vi "WaitOnSync.vi"(8 "error in (no error)":errorcluster, 9 "Enable":bool=TRUE, 11 "ControlState in":T1 {"ChainMask" format="0x%02x"}) -> (0 "error out":errorcluster, 3 "ControlState out":T1 {"ChainMask" format="0x%02x"})   [LabVIEW 2023, in "ArduinoSerialBling.lvlib"]
uses:
  ArduinoSerialBling.lvlib
  ControlState.ctl
  ConnectionType.ctl
  UdpConnection.ctl
  ChainState.ctl
  <vilib>/Instr/_visa.llb/VISA Flush IO Buffer Mask.ctl
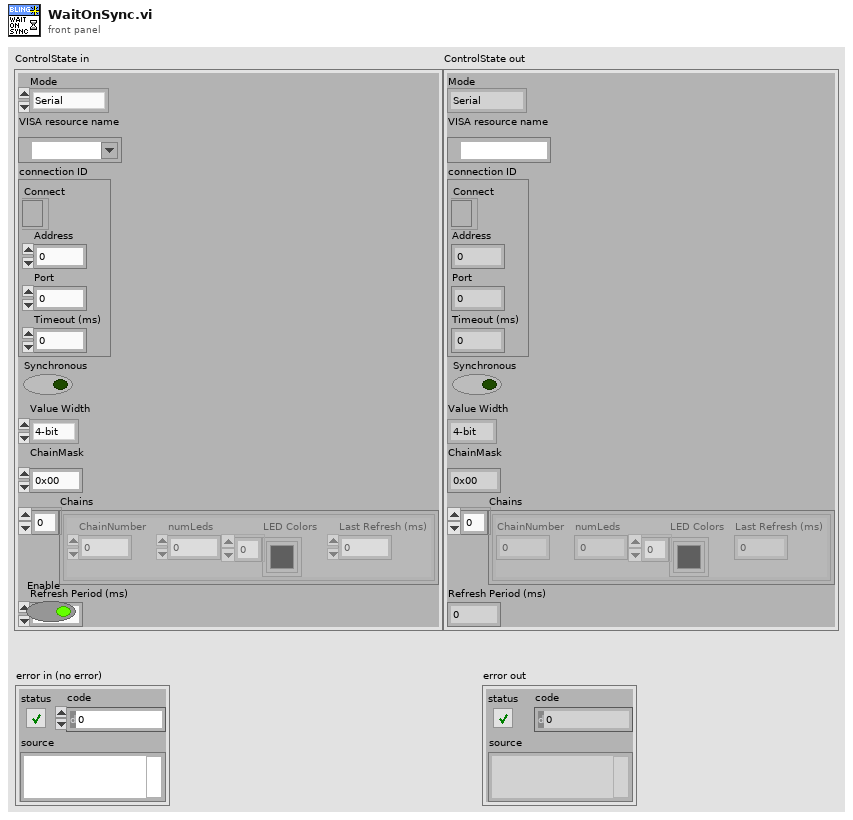
[diagram p1: front panel]
types:
  T1 = typedef "ArduinoSerialBling.lvlib/ControlState.ctl" = cluster{"Mode":T2, "VISA resource name":refnum<visa-resource-name>, "connection ID":T3, "Synchronous":bool, "Value Width":enum16{"4-bit", "8-bit"}, "ChainMask":u8, "Chains":T4[], "Refresh Period (ms)":u32}
  T2 = typedef "ConnectionType.ctl" = enum16{"Serial", "Ethernet", "Offline"}
  T3 = typedef "UdpConnection.ctl" = cluster{"Connect":refnum<k16>, "Address":u32, "Port":u16, "Timeout (ms)":i32}
  T4 = typedef "ArduinoSerialBling.lvlib/ChainState.ctl" = cluster{"ChainNumber":u8, "numLeds":u8, "LED Colors":u32[], "Last Refresh (ms)":u32}
  T5 = typedef "VISA Flush IO Buffer Mask.ctl" = u16
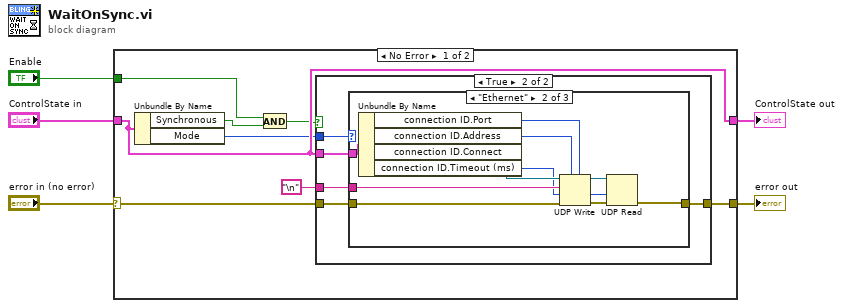
[diagram p0: block diagram]
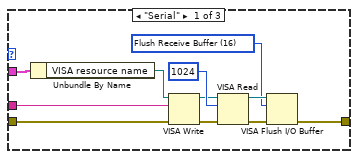
[diagram p3: hidden frame]
diagram:
  n1 = case shown="No Error" "error in (no error)" {
    selector: "error in (no error)" -> [w13 w43]
    tunnel: [w12 w43] -> w4
    tunnel: "ControlState in" -> [w11 w42]
    tunnel: [w11 w42] -> w2
    tunnel: "Enable" -> [w9 _]
    frame No Error {
      n2 = Unbundle By Name(w11) -> ("Synchronous"=w10:bool, "Mode"=w7:T2)
      n3 = And(x=w9, y=w10) -> (x .and. y?=w8:bool)
      n4 = case shown="True" w8 {
        tunnel: w13 -> [w14 w17]
        tunnel: [w14 w19] -> w12
        tunnel: w11 -> [_ w18]
        tunnel: w7 -> [_ w16]
        tunnel: "\n" -> [_ w15]
        frame False {
        }
        frame True {
          n5 = case shown="\"Ethernet\"" w16 {
            tunnel: [w27 w38 w41] -> w19
            tunnel: w18 -> [w25 w36 _]
            tunnel: w17 -> [w22 w40 w41]
            tunnel: w15 -> [w20 w37 _]
            frame "Serial" {
              w28 = T5 16 items=["Flush Receive Buffer"=16, "Write Transmit Buffer to Device"=32, "Flush Receive Buffer (No I/O)"=64, "Flush Transmit Buffer"=128] ("Mask")
              n6 = Unbundle By Name(w25) -> ("VISA resource name"=w24:refnum<visa-resource-name>)
              n7 = VISA Write(VISA resource name=w24, write buffer=w20, error in (no error)=w22) -> (VISA resource name out=w21:refnum<visa-resource-name>, error out=w23:errorcluster)  [unwired: 1 out]
              n8 = VISA Read(VISA resource name=w21, byte count=u32 1024, error in (no error)=w23) -> (VISA resource name out=w30:refnum<visa-resource-name>, error out=w29:errorcluster)  [unwired: 2 out]
              n9 = VISA Flush I/O Buffer(VISA resource name=w30, mask (16)=w28, error in (no error)=w29) -> (error out=w27:errorcluster)  [unwired: 1 out]
            }
            frame "Ethernet" {
              n10 = Unbundle By Name(w36) -> ("connection ID.Port"=w32:u16, "connection ID.Address"=w33:u32, "connection ID.Connect"=w35:refnum<k16>, "connection ID.Timeout (ms)"=w31:i32)
              n11 = UDP Write(address=w33, port or service name=w32, connection ID=w35, data in=w37, 8:w40, 9:w31) -> (error out=w39:errorcluster, 3:w34:refnum<k16>)
              n12 = UDP Read(connection ID=w34, timeout ms (25000)=w31, 8:w39) -> (error out=w38:errorcluster)  [unwired: 1 in, 4 out]
            }
            frame "Offline", Default {
            }
          }
        }
      }
    }
    frame Error {
    }
  }
  "ControlState out" <- w2
  "error out" <- w4
